vi "Start Sync.vi"(8 "error in (no error)":errorcluster, 11 "gRPC Server in":refnum<class "MeasurementService_Template.lvclass">) -> (0 "error out":errorcluster, 3 "gRPC Server out":refnum<class "MeasurementService_Template.lvclass">)   [LabVIEW 2020, in "LineRegulation.lvlib" / "MeasurementService_Template.lvclass"]
uses:
  MeasurementService_Template.lvclass
  MeasurementService_Template.lvclass/MeasurementService_Template.ctl
  RPC Messages/Measurement_v1_GetMetadataResponse/Measurement_v1_GetMetadataResponse_Data.ctl
  RPC Messages/Measurement_v1_MeasurementDetails/Measurement_v1_MeasurementDetails_Data.ctl
  RPC Messages/Measurement_v1_MeasurementParameters/Measurement_v1_MeasurementParameters_Data.ctl
  RPC Messages/Measurement_v1_ConfigurationParameter/Measurement_v1_ConfigurationParameter_Data.ctl
  RPC Messages/Measurement_v1_OutputParameter/Measurement_v1_OutputParameter_Data.ctl
  RPC Messages/Measurement_v1_UserInterfaceDetails/Measurement_v1_UserInterfaceDetails_Data.ctl
  Measurement Configuration.ctl
  RPC Messages/Measurement_v1_StopServiceResponse/Measurement_v1_StopServiceResponse_Data.ctl
  1b946eb2-f094-41b5-947e-49c608cc9ecf.vi
  d857de58-1d19-4099-89eb-555ae993dc53.vi
  <vilib>/gRPC/LabVIEW gRPC Library/Server API/Server/Get Server DLL Path.vi
  LineRegulation.lvlib
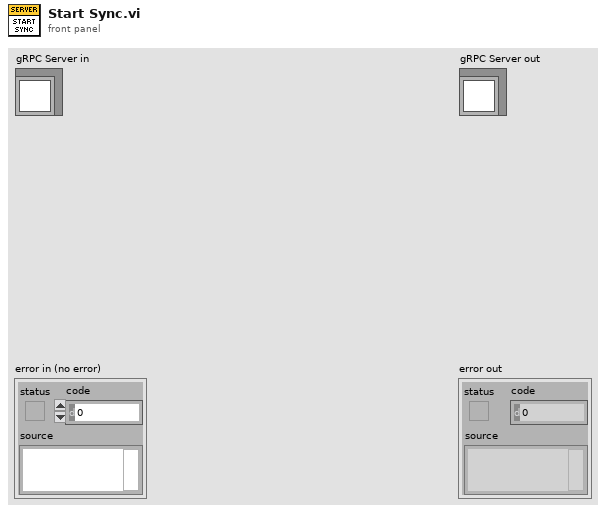
[diagram p1: front panel]
types:
  T1 = typedef "LineRegulation.lvlib/MeasurementService_Template.lvclass/Measurement_v1_GetMetadataResponse_Data.ctl" = cluster{"measurement_details":T2, "measurement_parameters":T3, "user_interface_details":T6}
  T2 = typedef "LineRegulation.lvlib/MeasurementService_Template.lvclass/Measurement_v1_MeasurementDetails_Data.ctl" = cluster{"display_name":string, "version":string, "measurement_type":string, "product_type":string}
  T3 = typedef "LineRegulation.lvlib/MeasurementService_Template.lvclass/Measurement_v1_MeasurementParameters_Data.ctl" = cluster{"configuration_parameters_messagetype":string, "configuration_parameters":T4[], "output_parameters_messagetype":string, "output_parameters":T5[]}
  T4 = typedef "LineRegulation.lvlib/MeasurementService_Template.lvclass/Measurement_v1_ConfigurationParameter_Data.ctl" = cluster{"protobuf_id":i32, "type":i32, "ArrayDimension":i32, "name":string, "parent":string}
  T5 = typedef "LineRegulation.lvlib/MeasurementService_Template.lvclass/Measurement_v1_OutputParameter_Data.ctl" = cluster{"protobuf_id":i32, "type":i32, "ArrayDimension":i32, "name":string, "parent":string}
  T6 = typedef "LineRegulation.lvlib/MeasurementService_Template.lvclass/Measurement_v1_UserInterfaceDetails_Data.ctl" = cluster{"configuration_ui_url":string}
  T7 = typedef "LineRegulation.lvlib/Measurement Configuration.ctl" = cluster{"Load Current in A":dbl, "Nominal Output Voltage in V":dbl, "Start":dbl, "Stop":dbl, "Step":dbl}
  T8 = typedef "LineRegulation.lvlib/MeasurementService_Template.lvclass/Measurement_v1_StopServiceResponse_Data.ctl" = cluster{"void":string}
  T9 = typedef "LineRegulation.lvlib/MeasurementService_Template.lvclass/Server gRPC UEs.ctl" = cluster{"Measurement_v1_MeasurementService_GetMetadata gRPC UE":refnum<user-event>, "Measurement_v1_MeasurementService_Measure gRPC UE":refnum<user-event>, "Measurement_v1_MeasurementService_StopService gRPC UE":refnum<user-event>}
  T10 = typedef "gprc-lvsupport-release.lvlib/grpcId.ctl" = u64
  T11 = typedef "LineRegulation.lvlib/MeasurementService_Template.lvclass/Measurement_v1_MeasureRequest_Data.ctl" = cluster{"configuration_arguments":T12}
  T12 = typedef "LineRegulation.lvlib/MeasurementService_Template.lvclass/google_protobuf_Any_Data.ctl" = cluster{"type_url":string, "value":u8[]}
  T13 = typedef "LineRegulation.lvlib/Measurement Results.ctl" = cluster{"Line Regulation (%/V)":dbl, "Line Regulation (%)":dbl, "Output Voltage in V":dbl[], "Test Results.Input Voltage in V":dbl[]}
  T14 = typedef "gprc-lvsupport-release.lvlib/Any.ctl" = cluster{"Type Url":string, "Bytes":u8[]}
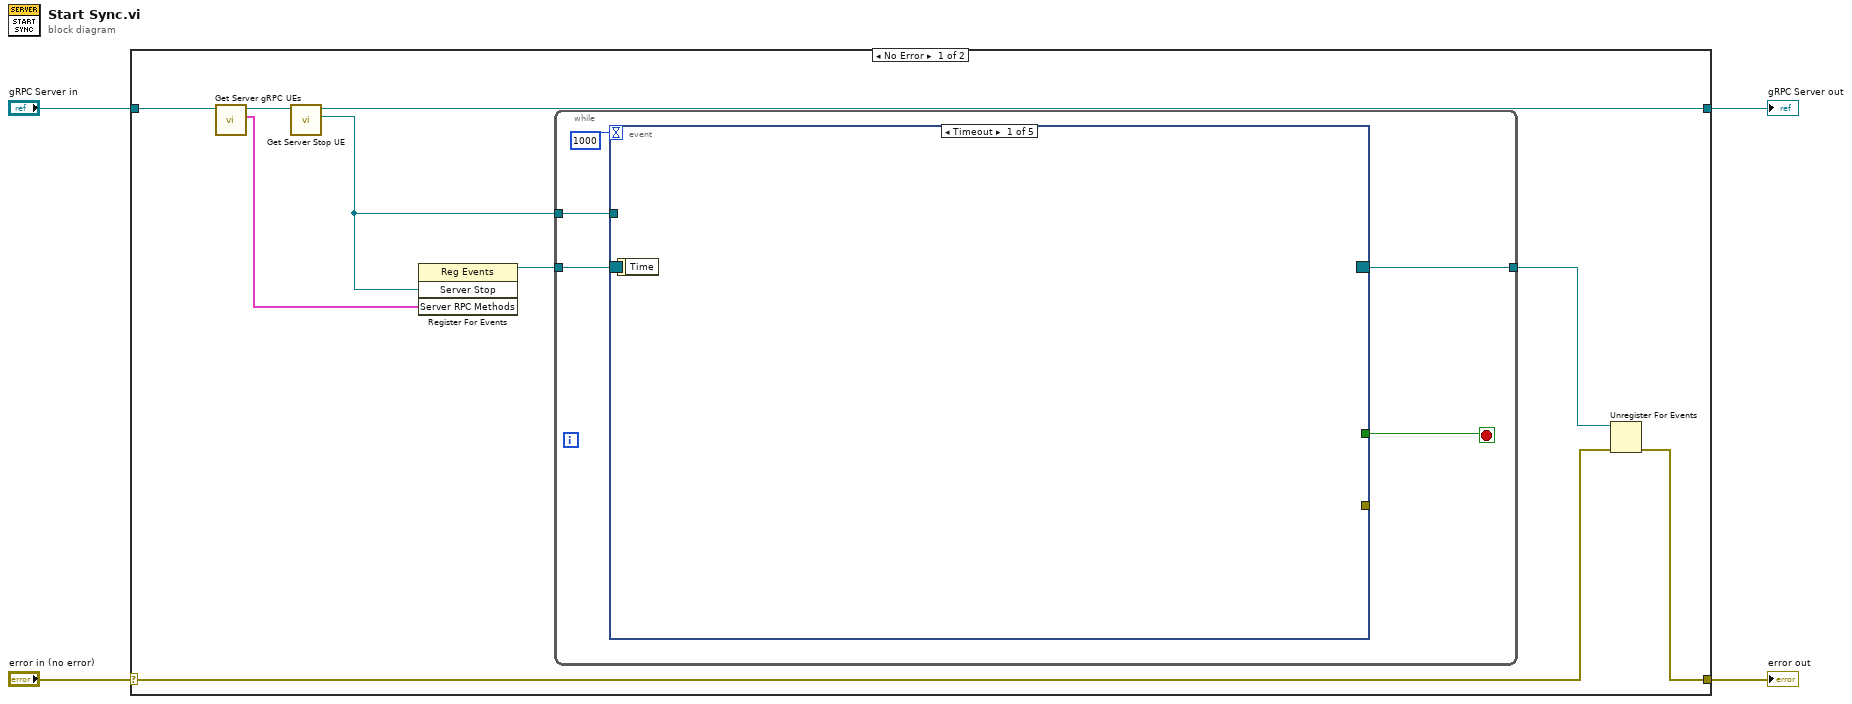
[diagram p0: block diagram]
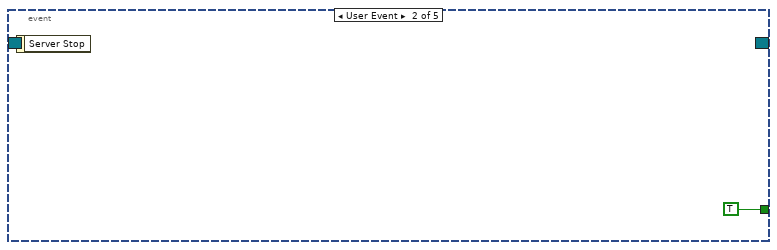
[diagram p2: hidden frame]
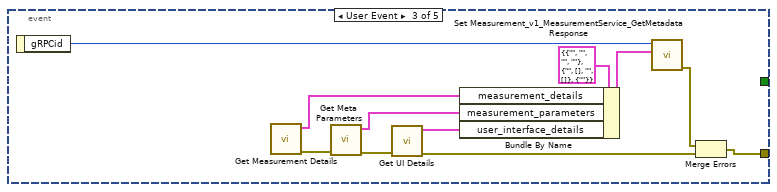
[diagram p3: hidden frame]
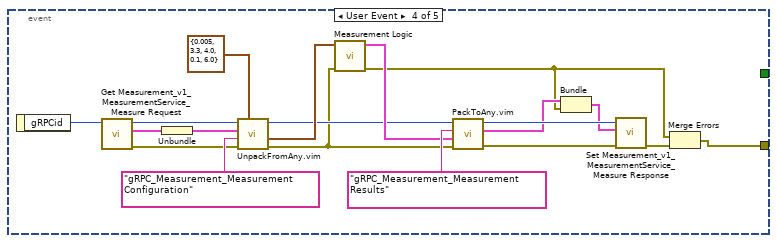
[diagram p4: hidden frame]
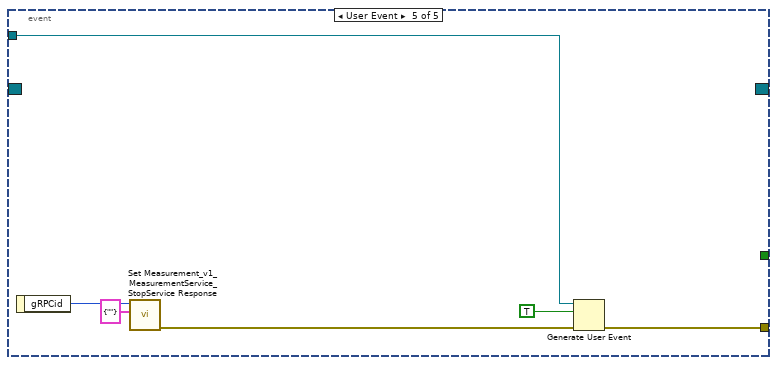
[diagram p5: hidden frame]
diagram:
  n1 = case shown="No Error" "error in (no error)" {
    selector: "error in (no error)" -> [w7 w57]
    tunnel: [w6 w57] -> w3
    tunnel: [w10 w56] -> w1
    tunnel: "gRPC Server in" -> [w13 w56]
    frame No Error {
      n2 = call "Get Server gRPC UEs.vi"("OOP Server in"=w13) -> ("Server RPC Methods"=w11:T9, "OOP Server out"=w12:refnum<class "MeasurementService_Template.lvclass">)  [unwired: 9 in]
      n3 = call "Get Server Stop UE.vi"("OOP Server in"=w12) -> ("Server Stop"=w5:refnum<user-event>, "OOP Server out"=w10:refnum<class "MeasurementService_Template.lvclass">)  [unwired: 9 in]
      n4 = register-events(w5, w11) -> (reference out=w9:refnum<event-registration>)  [unwired: 2 in, 1 out]
      n5 = while {
        tunnel: w9 -> [w18]
        tunnel: [w16] -> w8
        tunnel: w5 -> [w14]
        stop <- w17 stop-if-true
        n6 = event "RPC Methods Event Structure" shown="[0] Timeout" {
          selector: w18 -> [_ _ _ _ _]
          dyn-events: [_ _ _ _ _] -> w16
          timeout: 1000 -> [_ _ _ _ _]
          tunnel: [_ TRUE _ _ _] -> w17
          tunnel: [_ _ w21 w32 w54] -> _
          tunnel: w14 -> [_ _ _ _ w55]
          event Timeout {
            n7 = event-data() -> ()  [unwired: 1 in, 1 out]
          }
          event User Event {
            n8 = event-data() -> ()  [unwired: 1 in, 1 out]
          }
          event User Event {
            n9 = event-data() -> ("gRPCid"=w30:T10)  [unwired: 1 in]
            n10 = call "Get Measurement Details.vi"() -> ("error out"=w28:errorcluster, "measurement_details"=w26:T2)  [unwired: 10 in]
            n11 = call "Get Meta Parameters.vi"("error in"=w28) -> ("error out"=w29:errorcluster, "measurement_parameters"=w25:T3)  [unwired: 9 in]
            n12 = call "Get UI Details.vi"("error in"=w29) -> ("error out"=w23:errorcluster, "user_interface_details"=w24:T6)  [unwired: 9 in]
            n13 = Bundle By Name(cluster=T1 {"measurement_details"={"display_name"="", "version"="", "measurement_type"="", "product_type"=""}, "measurement_parameters"={"configuration_parameters_messagetype"="", "configuration_parameters"=[], "output_parameters_messagetype"="", "output_parameters"=[]}, "user_interface_details"={"configuration_ui_url"=""}} ("Message Data"), "measurement_details"=w26, "measurement_parameters"=w25, "user_interface_details"=w24) -> (w22:T1)
            n14 = call "Set Measurement_v1_MeasurementService_GetMetadata Response.vi"("Message Data"=w22, "gRPCid in"=w30) -> ("error out"=w20:errorcluster)  [unwired: 9 in]
            n15 = Merge Errors(w20, w23) -> (w21:errorcluster)
          }
          event User Event {
            n16 = event-data() -> ("gRPCid"=w42:T10)  [unwired: 1 in]
            n17 = call "Get Measurement_v1_MeasurementService_Measure Request.vi"("gRPCid in"=w42) -> ("error out"=w40:errorcluster, "Message Data"=w41:T11, "gRPCid out"=w36:T10)  [unwired: 8 in]
            n18 = Unbundle(w41) -> ("configuration_arguments"=w49:T12)
            n19 = call "UnpackFromAny.vim"("Data Type"=T7 {"Load Current in A"=0.005, "Nominal Output Voltage in V"=3.3, "Start"=4.0, "Stop"=0.1, "Step"=6.0} ("Measurement Configuration"), "error in (no error)"=w40, "Message Type"="gRPC_Measurement_Measurement Configuration", "Any"=w49, "gRPCid in"=w36) -> ("error out"=w37:errorcluster, "Unpacked Value"=w45:T7, "gRPCid"=w43:u64)  [unwired: 4 in]
            n20 = call "Measurement Logic.vi"("error in"=w37, "Measurement Configuration"=w45) -> ("error out"=w31:errorcluster, "Measurement Results"=w46:T13)  [unwired: 8 in]
            n21 = call "PackToAny.vim"("error in (no error)"=w37, "Data To Pack"=w46, "Message Type"="gRPC_Measurement_Measurement Results", "gRPCid in"=w43) -> ("error out"=w35:errorcluster, "Any"=w38:T14, "gRPCid"=w39:u64)  [unwired: 5 in]
            n22 = Bundle("Any"=w38, "error out"=w31) -> (w34:cluster{"Any":T14, "error out":errorcluster})  [unwired: 1 in]
            n23 = call "Set Measurement_v1_MeasurementService_Measure Response.vi"("error in (no error)"=w35, "Message Data"=w34, "gRPCid in"=w39) -> ("error out"=w33:errorcluster)  [unwired: 8 in]
            n24 = Merge Errors(w31, w33) -> (w32:errorcluster)
          }
          event User Event {
            n25 = event-data() -> ("gRPCid"=w52:T10)  [unwired: 1 in]
            n26 = call "Set Measurement_v1_MeasurementService_StopService Response.vi"("Message Data"=T8 {"void"=""}, "gRPCid in"=w52) -> ("error out"=w51:errorcluster)  [unwired: 9 in]
            n27 = Generate User Event(user event=w55, event data cluster=TRUE ("event data"), error in=w51) -> (error out=w54:errorcluster)  [unwired: 1 in, 1 out]
          }
        }
      }
      n28 = Unregister For Events(event registration refnum=w8, error in=w7) -> (error out=w6:errorcluster)
    }
    frame Error {
    }
  }
  "error out" <- w3
  "gRPC Server out" <- w1
